vi "Table_CellValue_Tests.vi"(8 "error in":errorcluster) -> (0 "error out":errorcluster)   [LabVIEW 2016, in "DronaTest.lvlib"]
uses:
  DronaTest.lvlib
  APIs/Stimulus/ControlValue/SetValueAuto.vi
  APIs/Stimulus/ControlValue/Controls/Table/EditCellValue.vi
  APIs/Assert/AssertControlValue/Controls/Table/AssertCellValue.vi
  <vilib>/addons/_JKI Toolkits/Caraya/classes/Assert/Assert Error.vi
  <vilib>/addons/_JKI Toolkits/Caraya/classes/Test/Test.lvclass
  <vilib>/SLL Toolkit/SLL Debug/SLL Debug.lvlib
  Drona.lvlib
  <vilib>/addons/_JKI Toolkits/Caraya/classes/Assert/Assert.lvclass
  APIs/Stimulus/ControlValue/Controls/Table/StimulusTable.lvlib
  APIs/Assert/AssertControlValue/Controls/Table/AssertTable.lvlib
  APIs/Stimulus/ControlValue/ControlValue.lvlib
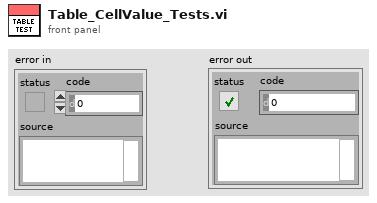
[diagram p1: front panel]
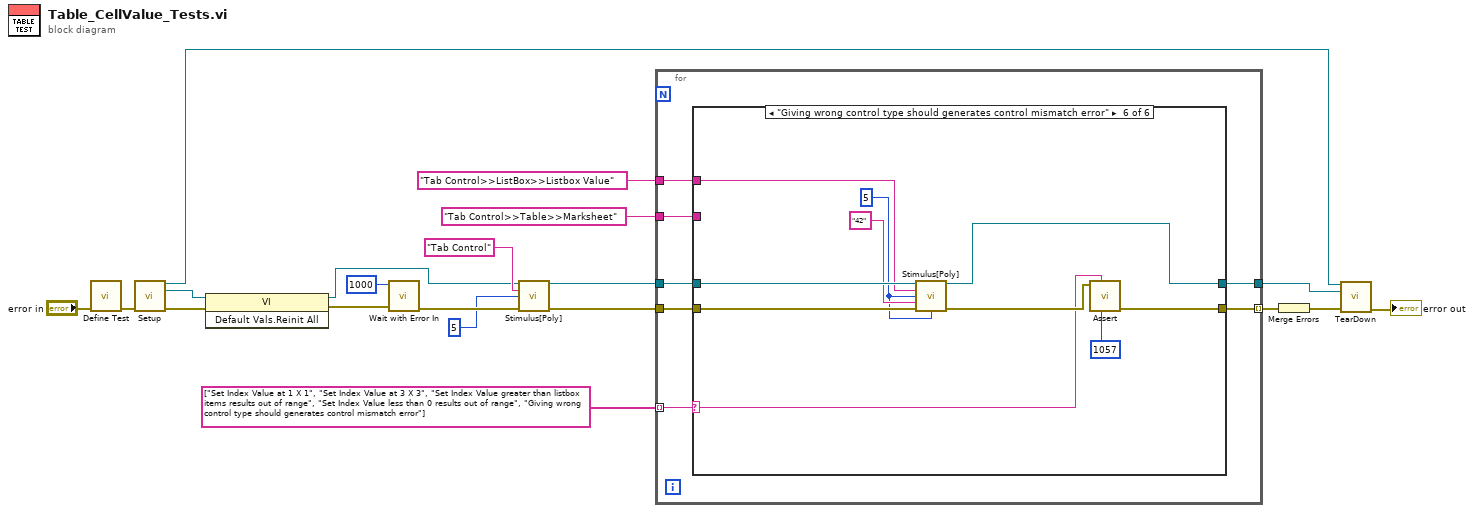
[diagram p0: block diagram]
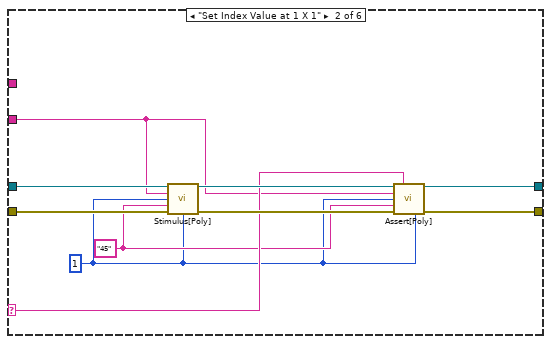
[diagram p3: hidden frame]
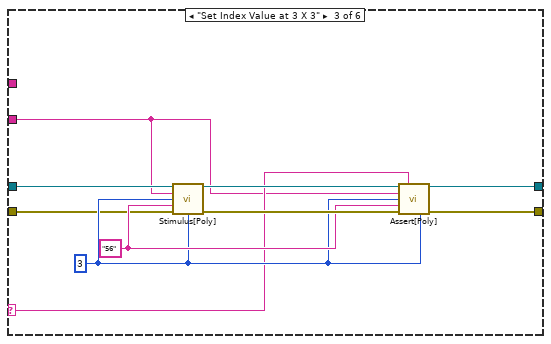
[diagram p4: hidden frame]
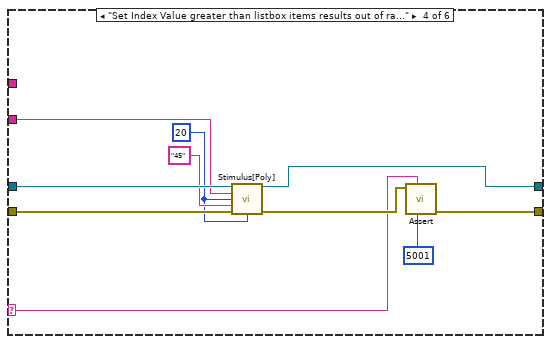
[diagram p5: hidden frame]
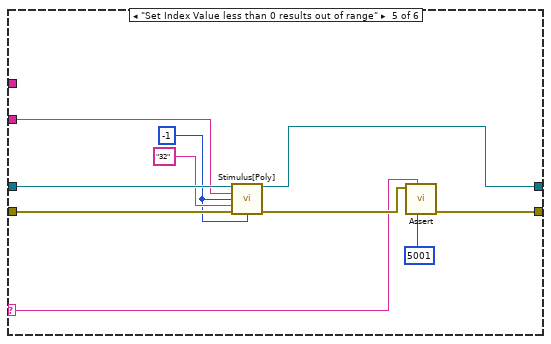
[diagram p6: hidden frame]
diagram:
  n1 = call <vilib>:"Define Test.vi"("error in (no error)"="error in") -> ("error out"=w10:errorcluster)  [unwired: 9 in, 1 out]
  n2 = call "Setup.vi"("error in (no error)"=w10) -> ("Application Ref"=w8:refnum<vi>, "VI out"=w2:refnum<vi>, "error out"=w4:errorcluster)  [unwired: 12 in]
  n3 = invoke class="VI" method="Default Vals.Reinit All"(reference=w2, error in=w4) -> (reference out=w1:refnum<vi>, error out=w3:errorcluster)  [unwired: 1 in, 1 out]
  n4 = call <vilib>:"Wait with Error In.vi"("error in (no error)"=w3, "milliseconds to wait"=u32 1000) -> ("error out"=w18:errorcluster)  [unwired: 9 in]
  n5 = call-poly "Stimulus[Poly].vi"("VI Reference In"=w1, "Control Path"="Tab Control", "Value (Signaling)"=5, "error in"=w18) -> ("VI Reference Out"=w14:refnum<vi>, "error out"=w17:errorcluster)  [unwired: 10 in]
  n6 = for {
    tunnel: w14 -> [w26]
    tunnel: "Tab Control>>Table>>Marksheet" ("Control Path") -> [w25]
    tunnel: "Tab Control>>ListBox>>Listbox Value" ("Control Path") -> [w24]
    tunnel: string[] ["Set Index Value at 1 X 1", "Set Index Value at 3 X 3", "Set Index Value greater than listbox items results out of range", "Set Index Value less than 0 results out of range", "Giving wrong control type should generates control mismatch error"] -> [w22] mode=indexing
    tunnel: [w21] -> w7
    tunnel: w17 -> [w27]
    tunnel: [w23] -> w11 mode=indexing
    n7 = case shown="\"Giving wrong control type should generates control mismatch error\"" w22 {
      selector: w22 -> [_ w33 w41 w54 w64 w75]
      tunnel: w27 -> [w29 w39 w44 w59 w69 w79]
      tunnel: w26 -> [w28 w38 w45 w58 w68 w78]
      tunnel: w25 -> [_ w30 w40 w57 w67 _]
      tunnel: w24 -> [_ _ _ _ _ w72]
      tunnel: [w29 w35 w42 w55 w65 w76] -> w23
      tunnel: [w28 w34 w43 w52 w62 w73] -> w21
      frame Default {
      }
      frame "Set Index Value at 1 X 1" {
        w32 = "45" ("Value")
        w31 = 1 ("Item Index")
        n8 = call-poly "Stimulus[Poly].vi"("VI Reference In"=w38, "Control Path"=w30, "Row Index"=w31, "Value"=w32, "Error In"=w39, "Column Index"=w31) -> ("VI Reference Out"=w36:refnum<vi>, "Error Out"=w37:errorcluster)  [unwired: 8 in]
        n9 = call-poly "Assert[Poly].vi"("VI Reference In"=w36, "Test Label"=w33, "Control Path"=w30, "Row Index"=w31, "Item Value"=w32, "Error In"=w37, "Column Index"=w31) -> ("VI Reference Out"=w34:refnum<vi>, "Error Out"=w35:errorcluster)  [unwired: 6 in, 1 out]
      }
      frame "Set Index Value at 3 X 3" {
        w47 = "56" ("Value")
        w46 = 3 ("Item Index")
        n10 = call-poly "Stimulus[Poly].vi"("VI Reference In"=w45, "Control Path"=w40, "Row Index"=w46, "Value"=w47, "Error In"=w44, "Column Index"=w46) -> ("VI Reference Out"=w48:refnum<vi>, "Error Out"=w49:errorcluster)  [unwired: 8 in]
        n11 = call-poly "Assert[Poly].vi"("VI Reference In"=w48, "Test Label"=w41, "Control Path"=w40, "Row Index"=w46, "Item Value"=w47, "Error In"=w49, "Column Index"=w46) -> ("VI Reference Out"=w43:refnum<vi>, "Error Out"=w42:errorcluster)  [unwired: 6 in, 1 out]
      }
      frame "Set Index Value greater than listbox items results out of range" {
        w50 = 20 ("Item Index")
        n12 = call-poly "Stimulus[Poly].vi"("VI Reference In"=w58, "Control Path"=w57, "Row Index"=w50, "Value"="45", "Error In"=w59, "Column Index"=w50) -> ("VI Reference Out"=w52:refnum<vi>, "Error Out"=w56:errorcluster)  [unwired: 8 in]
        n13 = call-poly <vilib>:"Assert.vi"("error code (1)"=5001, "Label"=w54, "Error?"=w56) -> ("error out"=w55:errorcluster)  [unwired: 7 in, 1 out]
      }
      frame "Set Index Value less than 0 results out of range" {
        w60 = -1 ("Item Index")
        n14 = call-poly "Stimulus[Poly].vi"("VI Reference In"=w68, "Control Path"=w67, "Row Index"=w60, "Value"="32", "Error In"=w69, "Column Index"=w60) -> ("VI Reference Out"=w62:refnum<vi>, "Error Out"=w66:errorcluster)  [unwired: 8 in]
        n15 = call-poly <vilib>:"Assert.vi"("error code (1)"=5001, "Label"=w64, "Error?"=w66) -> ("error out"=w65:errorcluster)  [unwired: 7 in, 1 out]
      }
      frame "Giving wrong control type should generates control mismatch error" {
        w70 = 5 ("Item Index")
        n16 = call-poly "Stimulus[Poly].vi"("VI Reference In"=w78, "Control Path"=w72, "Row Index"=w70, "Value"="42", "Error In"=w79, "Column Index"=w70) -> ("VI Reference Out"=w73:refnum<vi>, "Error Out"=w77:errorcluster)  [unwired: 8 in]
        n17 = call-poly <vilib>:"Assert.vi"("error code (1)"=1057, "Label"=w75, "Error?"=w77) -> ("error out"=w76:errorcluster)  [unwired: 7 in, 1 out]
      }
    }
  }
  n18 = Merge Errors(w11) -> (w9:errorcluster)
  n19 = call "TearDown.vi"("Application Ref"=w8, "VI in"=w7, "error in (no error)"=w9) -> ("error out"=→"error out":errorcluster)  [unwired: 12 in]
